vi "Load Hardware Config.vi"(8 "error in":errorcluster, 11 "Config path":path=path "C:/GitHub/GIP-FCT/Config/Hardware Config.ini") -> (0 "error out":errorcluster)   [LabVIEW 2021]
uses:
  Controls/DAQ_Data.ctl
  Controls/Instruments_Data.ctl
  Controls/MUX_Data.ctl
  Controls/DMM_Data.ctl
  <vilib>/Utility/config.llb/Read Key (String).vi
  <vilib>/Utility/config.llb/NI_LVConfig.lvlib
panel:
  out "data":T1[](array[typedef])
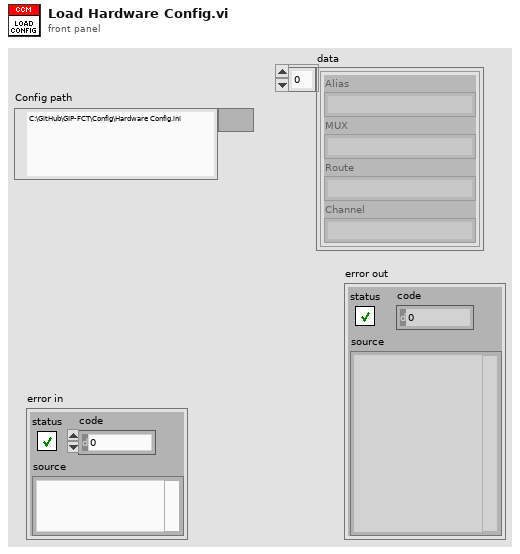
[diagram p1: front panel]
types:
  T1 = typedef "DAQ_Data.ctl" = cluster{"Alias":string, "MUX":string, "Route":string, "Channel":string}
  T2 = typedef "NI_LVConfig.lvlib/Config Data RefNum.ctl" = refnum<k1>
  T3 = typedef "Instruments_Data.ctl" = cluster{"Alias":string, "Resource ":string}
  T4 = typedef "MUX_Data.ctl" = cluster{"Alias":string, "Topology":string}
  T5 = typedef "DMM_Data.ctl" = cluster{"Alias":string, "MUX":string, "Route":string}
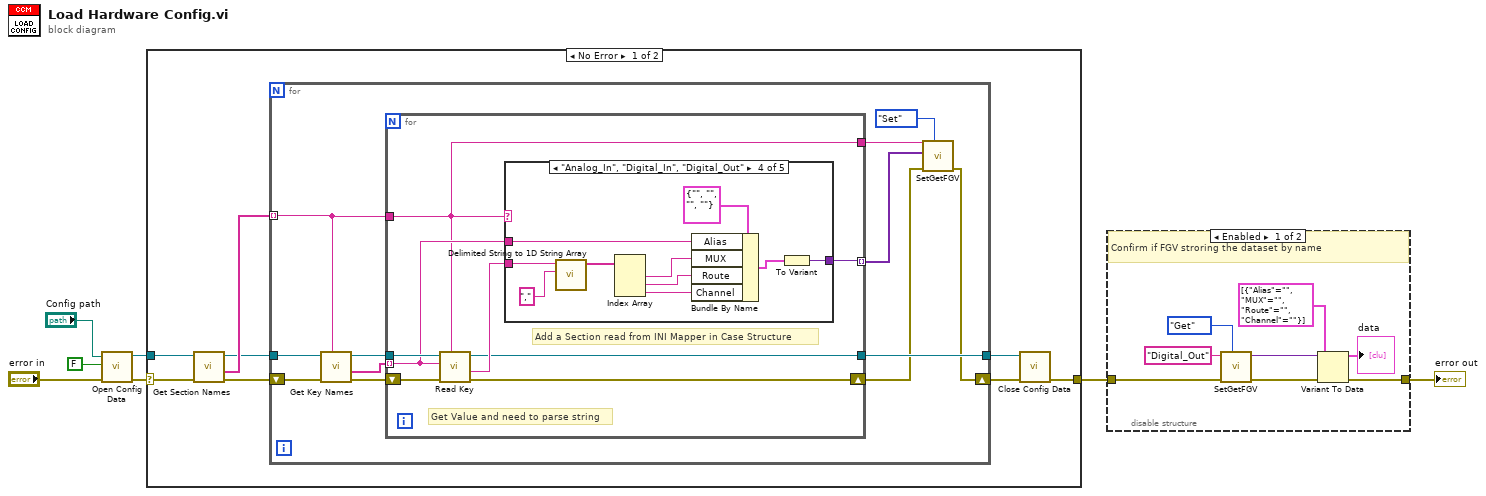
[diagram p0: block diagram]
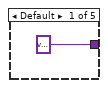
[diagram p2: hidden frame]
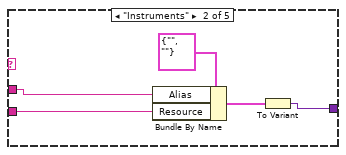
[diagram p3: hidden frame]
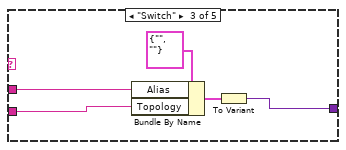
[diagram p4: hidden frame]
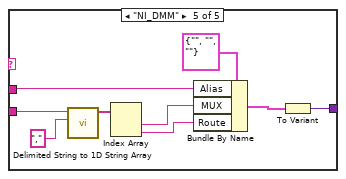
[diagram p5: hidden frame]
diagram:
  n1 = call <vilib>:"Open Config Data.vi"("error in (no error)"="error in", "create file if necessary (T)"=FALSE, "configuration file path"="Config path") -> ("error out"=w5:errorcluster, "refnum"=w6:T2)  [unwired: 6 in, 1 out]
  n2 = case shown="No Error" w5 {
    selector: w5 -> [w15 w66]
    tunnel: [w8 w66] -> w2
    tunnel: w6 -> [w14 _]
    frame No Error {
      n3 = call <vilib>:"Get Section Names.vi"("error in (no error)"=w15, "refnum"=w14) -> ("error out"=w12:errorcluster, "section names"=w13:string[], "refnum out"=w11:T2)  [unwired: 7 in]
      n4 = for {
        tunnel: w13 -> [w24] mode=indexing
        tunnel: w11 -> [w26]
        tunnel: [w25] -> w10
        shift-right: [w17] -> w9
        shift-left: w12 -> [w27]
        n5 = call <vilib>:"Get Key Names.vi"("section"=w24, "error in (no error)"=w27, "refnum"=w26) -> ("error out"=w23:errorcluster, "key names"=w22:string[], "refnum out"=w21:T2)  [unwired: 5 in, 1 out]
        n6 = for {
          tunnel: w22 -> [w32] mode=indexing
          tunnel: w24 -> [w28]
          tunnel: w21 -> [w34]
          tunnel: [w30] -> w25
          tunnel: [w29] -> w19 mode=indexing
          shift-right: [w33] -> w18
          shift-left: w23 -> [w35]
          tunnel: [w28] -> w16
          # "Add a Section read from INI Mapper in Case Structure"
          # "Get Value and need to parse string"
          n7 = call-poly <vilib>:"Read Key.vi"("section"=w28, "error in (no error)"=w35, "key"=w32, "refnum"=w34) -> ("error out"=w33:errorcluster, "value"=w31:string, "refnum out"=w30:T2)  [unwired: 4 in, 1 out]
          n8 = case shown="\"Analog_In\", \"Digital_In\", \"Digital_Out\"" w28 {
            tunnel: w32 -> [_ w39 w45 w52 w59]
            tunnel: w31 -> [_ w40 w44 w53 w60]
            tunnel: [variant ("Variant") w38 w43 w48 w58] -> w29
            frame Default {
            }
            frame "Instruments" {
              n9 = Bundle By Name(cluster=T3 {"Alias"="", "Resource "=""} ("Instruments Data"), "Alias"=w39, "Resource"=w40) -> (w41:T3)
              n10 = To Variant(anything=w41) -> (Variant=w38:variant)
            }
            frame "Switch" {
              n11 = Bundle By Name(cluster=T4 {"Alias"="", "Topology"=""}, "Alias"=w45, "Topology"=w44) -> (w42:T4)
              n12 = To Variant(anything=w42) -> (Variant=w43:variant)
            }
            frame "Analog_In", "Digital_In", "Digital_Out" {
              n13 = call <vilib>:"Delimited String to 1D String Array.vi"("delimiter"=",", "delimited string"=w53) -> ("string array"=w51:string[])  [unwired: 9 in]
              n14 = Index Array(array=w51) -> (element #1=w55:string, element #2=w54:string, element #3=w47:string)  [unwired: 3 in]
              n15 = Bundle By Name(cluster=T1 {"Alias"="", "MUX"="", "Route"="", "Channel"=""} ("DAQ Data"), "Alias"=w52, "MUX"=w55, "Route"=w54, "Channel"=w47) -> (w49:T1)
              n16 = To Variant(anything=w49) -> (Variant=w48:variant)
            }
            frame "NI_DMM" {
              n17 = call <vilib>:"Delimited String to 1D String Array.vi"("delimiter"=",", "delimited string"=w60) -> ("string array"=w61:string[])  [unwired: 9 in]
              n18 = Index Array(array=w61) -> (element #1=w64:string, element #2=w65:string)  [unwired: 2 in]
              n19 = Bundle By Name(cluster=T5 {"Alias"="", "MUX"="", "Route"=""} ("DMM Data"), "Alias"=w59, "MUX"=w64, "Route"=w65) -> (w63:T5)
              n20 = To Variant(anything=w63) -> (Variant=w58:variant)
            }
          }
        }
        n21 = call "SetGetFGV.vi"("Method (Get)"=enum16{"Get", "Set"}."Set", "error in"=w18, "Data In"=w19, "FGVname"=w16) -> ("error out"=w17:errorcluster)  [unwired: 6 in, 1 out]
      }
      n22 = call <vilib>:"Close Config Data.vi"("error in (no error)"=w9, "refnum"=w10) -> ("error out"=w8:errorcluster)  [unwired: 8 in, 1 out]
    }
    frame Error {
    }
  }
  n23 = disable-structure "Diagram Disable Structure" shown="Enabled" {
    disable-tunnel: w2 -> [w74 w75]
    disable-tunnel: [w70 w75] -> w1
    frame Enabled {
      # "Confirm if FGV stroring the dataset by name"
      n24 = call "SetGetFGV.vi"("Method (Get)"=enum16{"Get", "Set"}."Get", "error in"=w74, "FGVname"="Digital_Out") -> ("error out"=w72:errorcluster, "Data out"=w71:variant)  [unwired: 7 in]
      n25 = Variant To Data(error in=w72, type=T1[] [{"Alias"="", "MUX"="", "Route"="", "Channel"=""}], Variant=w71) -> (data=→"data":T1[], error out=w70:errorcluster)
    }
    frame Disabled {
    }
  }
  "error out" <- w1
